vi "Counter Preset.vi"(7 "Read Value? (F)":bool, 8 "error in (no error)":errorcluster, 9 "Counter Preset (1)":u64=1 min=1 max=900000000000 step=1 format="%#_1e", 10 "Counter (T)":T1=enum."T", 11 "VISA resource name":refnum<visa-resource-name>) -> (0 "error out":errorcluster, 1 "Counter Preset":u64=1 format="%.0e", 3 "VISA resource name out":refnum<visa-resource-name>)   [LabVIEW 2013, in "SRS SR400.lvlib"]
doc: "<B>CP i { ,n }</B>\n\nThe CP command sets and reads the counter presets. If i = 1 then counter B is selected, if i = 2 counter T is selected. The parameter i is required. If n is included, then counter i is preset to n where n is a value from 1 to 9E11. n may be expressed in any format but must be greater than or equal to 1 and only the most significant digit is used. For example, \"CP2,10\" , \"CP2,1E1\" , \"CP2,0.1E2\", \"CP2,12\" all set T SET to 1E1. Changing a counter preset while counting causes the counters to pause. A counter start command or keypress resumes counting. If n is absent, then the preset value of counter i is returned. In the above example, the string \"1E1\" is returned. Note that n is the number of cycles of the 10 MHz clock, not seconds."
uses:
  <instrlib>/SRS SR400/SRS SR400.lvlib
  <instrlib>/SRS SR400/Public/Typedefs/Counter (Preset).ctl
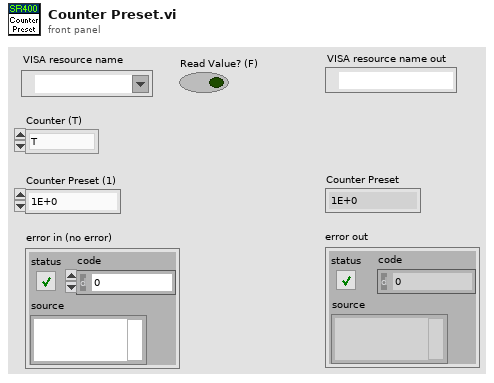
[diagram p1: front panel]
types:
  T1 = typedef "SRS SR400.lvlib/Counter (Preset).ctl" = enum16{"Invalid", "B", "T"}
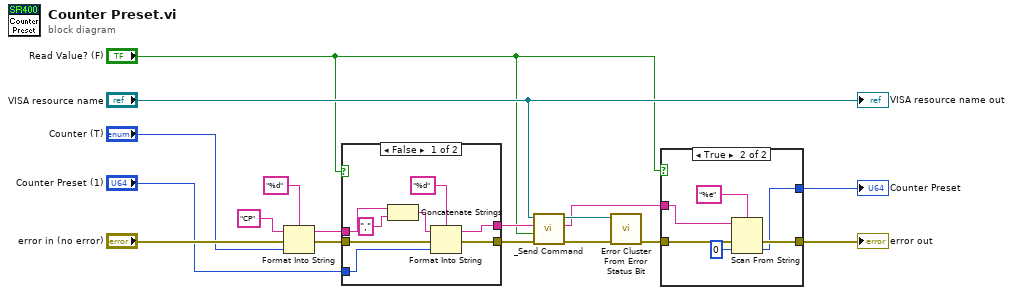
[diagram p0: block diagram]
diagram:
  n1 = Format Into String(format string="%d", initial string="CP" ("command"), error in="error in (no error)", "Counter (T)") -> (resulting string=w15:string, error out=w16:errorcluster)
  n2 = case shown="False" "Read Value? (F)" {
    tunnel: w16 -> [w25 w26]
    tunnel: w15 -> [w24 w27]
    tunnel: "Counter Preset (1)" -> [w18 _]
    tunnel: [w20 w27] -> w10
    tunnel: [w19 w26] -> w9
    frame False {
      n3 = Concatenate Strings(w24, "," ("command")) -> (w22:string)
      n4 = Format Into String(format string="%d", initial string=w22, error in=w25, w18) -> (resulting string=w20:string, error out=w19:errorcluster)
    }
    frame True {
    }
  }
  n5 = call <instrlib>:"_Send Command.vi"("error in (no error)"=w9, "Read Value? (F)"="Read Value? (F)", "Command"=w10, "VISA resource name"="VISA resource name") -> ("error out"=w6:errorcluster, "Response"=w2:string, "VISA resource name out"=w7:refnum<visa-resource-name>)  [unwired: 5 out]
  n6 = call <instrlib>:"Error Cluster From Error Status Bit.vi"("error in (no error)"=w6, "VISA resource name"=w7) -> ("error out"=w5:errorcluster)  [unwired: 8 in, 1 out]
  n7 = case shown="True" "Read Value? (F)" {
    tunnel: w5 -> [w28 w34]
    tunnel: [w28 w33] -> w4
    tunnel: w2 -> [_ w31]
    tunnel: [_ w29] -> w1
    frame False {
    }
    frame True {
      n8 = Scan From String(format string="%e", input string=w31, error in=w34, default 1=u64 0 ("default value 1")) -> (error out=w33:errorcluster, output 1=w29:u64)  [unwired: 1 in, 2 out]
    }
  }
  "error out" <- w4
  "Counter Preset" <- w1
  "VISA resource name out" <- "VISA resource name"
